vi "scan2d_get_duration.vi"(7 "current_iteration":u32, 8 "error in (no error)":errorcluster, 9 "current_y":dbl, 10 "current_x":dbl, 11 "scan_panel in":refnum<class "scan_2d.lvclass">) -> (0 "error out":errorcluster, 2 "time_remaining":string, 3 "scan_panel out":refnum<class "scan_2d.lvclass">)   [LabVIEW 2015, in "scan_2d.lvclass"]
uses:
  scan_2d.lvclass
  scan_2d.lvclass/scan_2d.ctl
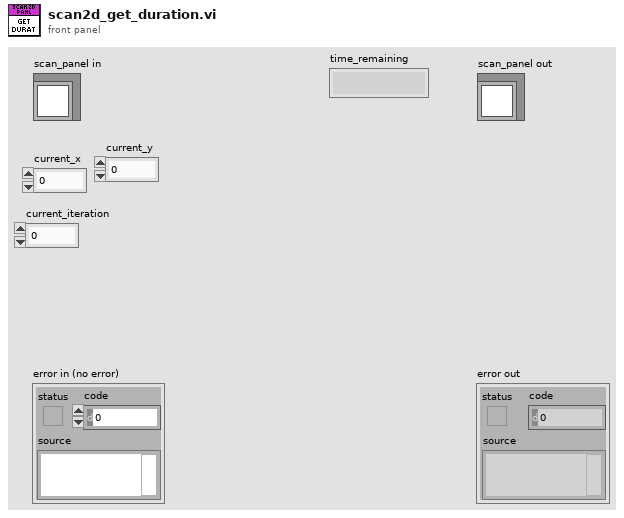
[diagram p1: front panel]
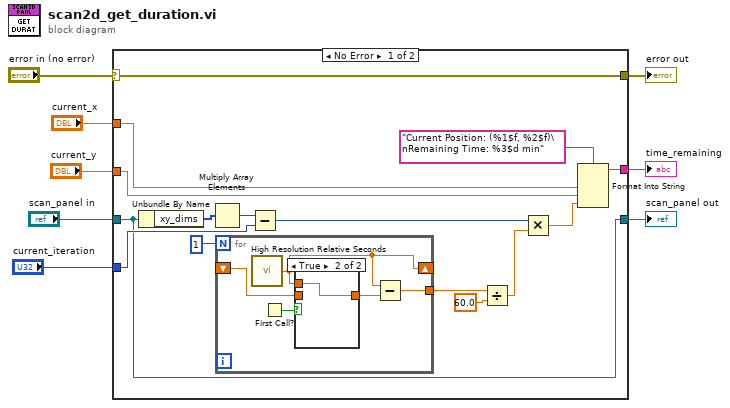
[diagram p0: block diagram]
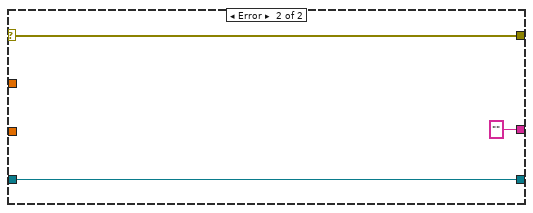
[diagram p3: hidden frame]
diagram:
  n1 = case shown="No Error" "error in (no error)" {
    selector: "error in (no error)" -> [w23 w33]
    tunnel: [w23 w33] -> w7
    tunnel: [w11 w32] -> w5
    tunnel: "scan_panel in" -> [w11 w32]
    tunnel: "current_x" -> [w14 _]
    tunnel: "current_iteration" -> [w18 _]
    tunnel: [w15 ""] -> w2
    tunnel: "current_y" -> [w13 _]
    frame No Error {
      n2 = Unbundle By Name(w11) -> ("xy_dims"=w10:u32[])
      n3 = Multiply Array Elements(1:w10) -> (0:w9:u32)
      n4 = for {
        N: 1 -> [_]
        shift-right: [w25] -> _
        shift-left: _ -> [w27]
        tunnel: [w28] -> w20
        n5 = call <vilib>:"High Resolution Relative Seconds.vi"() -> ("relative seconds"=w25:dbl)
        n6 = First Call?() -> (First Call?: T/F=w24:bool)
        n7 = case shown="True" w24 {
          tunnel: w27 -> [w29 _]
          tunnel: [w29 w30] -> w26
          tunnel: w25 -> [_ w30]
          frame False {
          }
          frame True {
          }
        }
        n8 = Subtract(x=w25, y=w26) -> (x-y=w28:dbl)
      }
      n9 = Subtract(x=w9, y=w18) -> (x-y=w17:u32)
      n10 = Divide(x=w20, y=60.0) -> (x/y=w16:dbl)
      n11 = Multiply(x=w17, y=w16) -> (x*y=w12:dbl)
      n12 = Format Into String(format string="Current Position: (%1$f, %2$f)\nRemaining Time: %3$d min", w14, w13, w12) -> (resulting string=w15:string)  [unwired: 2 in, 1 out]
    }
    frame Error {
    }
  }
  "error out" <- w7
  "scan_panel out" <- w5
  "time_remaining" <- w2
